vi "CNC.vi"(6 "pause":bool, 7 "start":bool, 8 "products in":u16, 9 "speed in":i32(listbox), 10 "Thermometer in":dbl(slide) scale=0.0..100.0, 11 "speed in":dbl(knob) scale=0.0..10.0) -> (0 "products out":u16, 2 "Thermometer out":dbl(slide) scale=0.0..100.0, 3 "speed out":dbl(knob) scale=0.0..10.0)   [LabVIEW 2026]
uses:
  <vilib>/numeric/Random Number (Range) DBL.vi
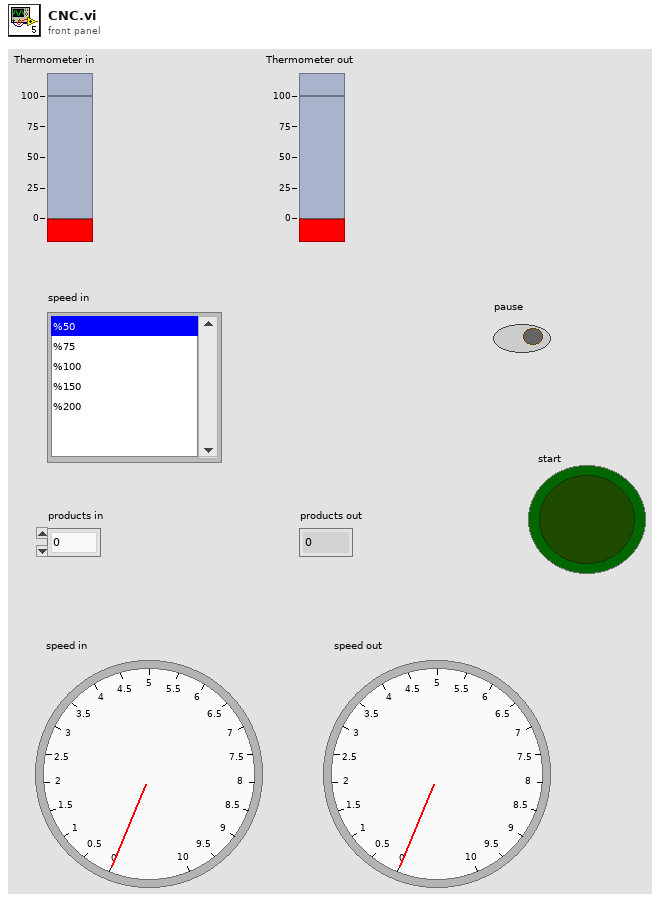
[diagram p1: front panel]
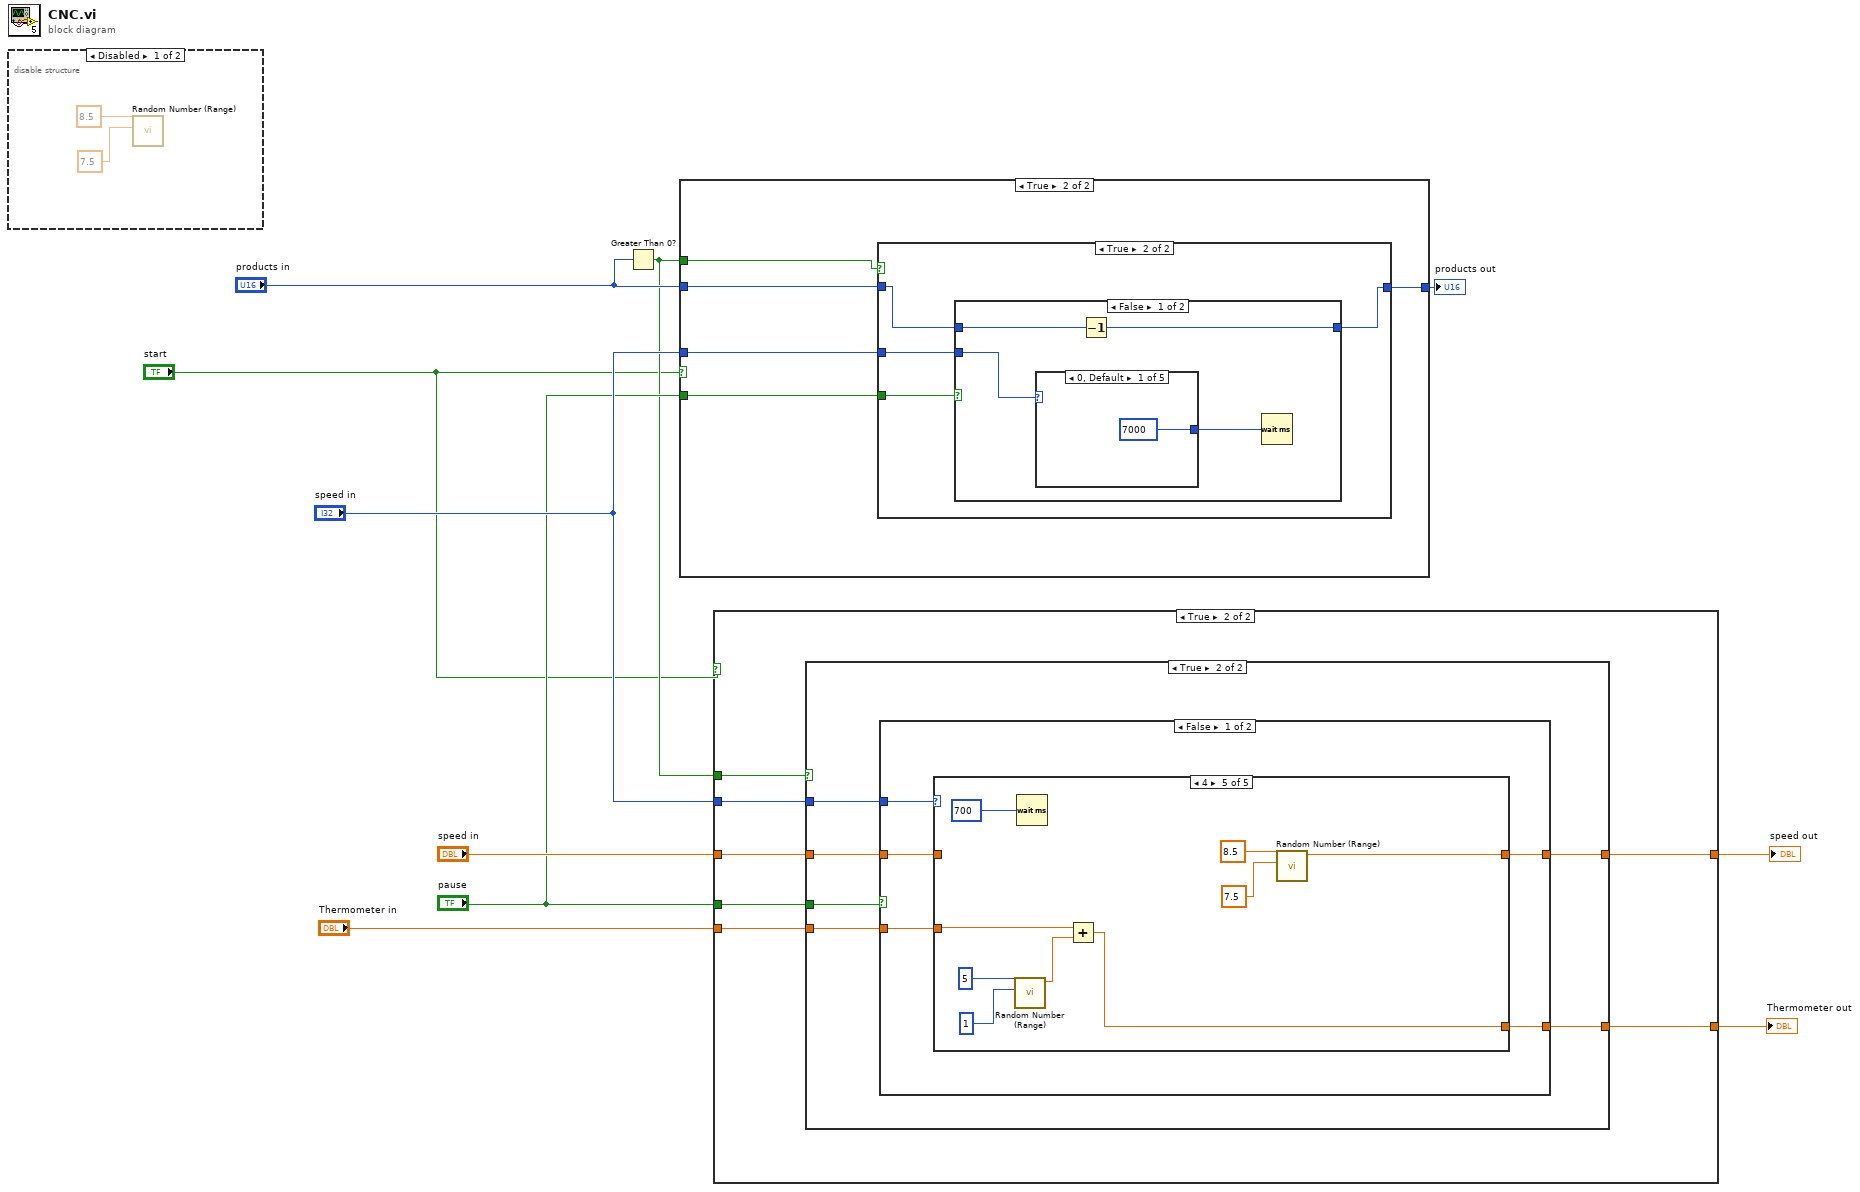
[diagram p0: block diagram]
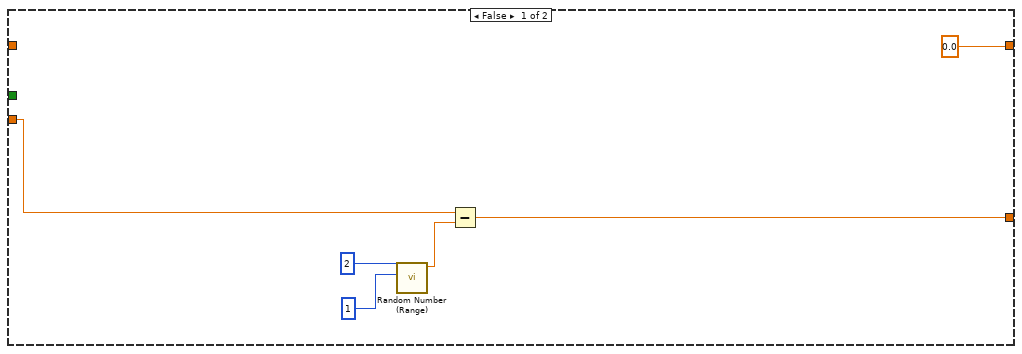
[diagram p2: hidden frame]
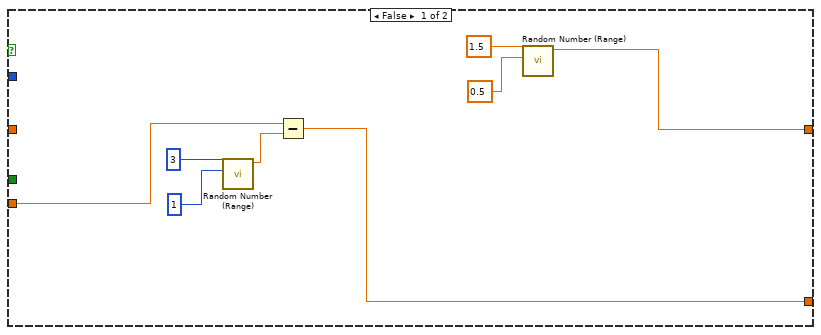
[diagram p3: hidden frame]
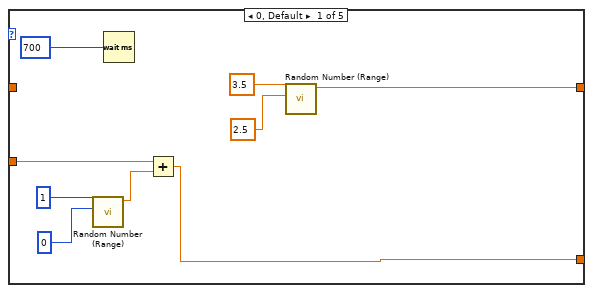
[diagram p4: hidden frame]
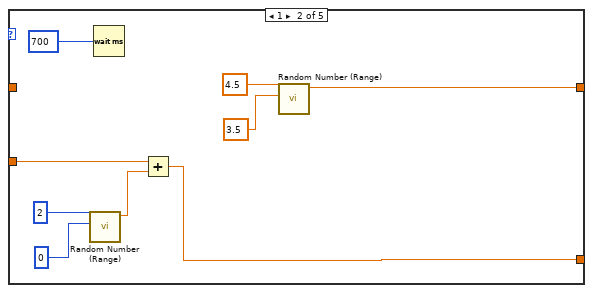
[diagram p5: hidden frame]
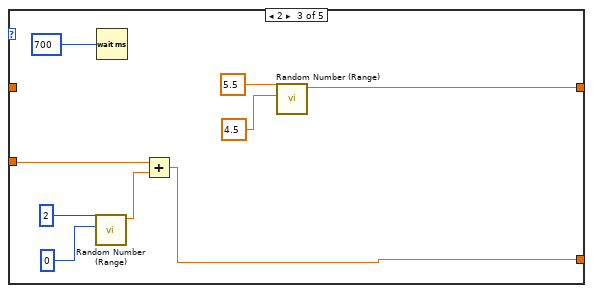
[diagram p6: hidden frame]
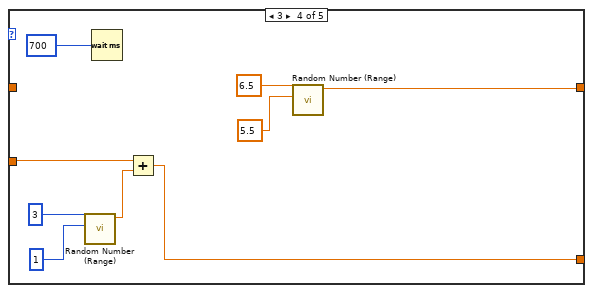
[diagram p7: hidden frame]
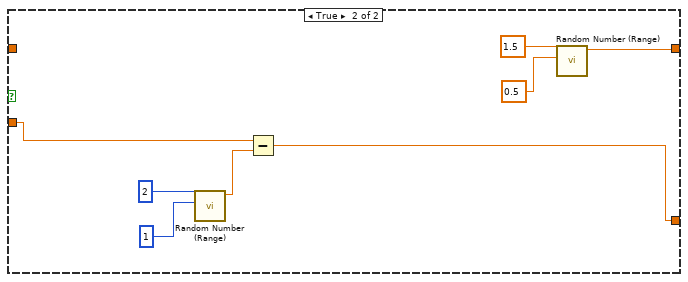
[diagram p8: hidden frame]
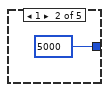
[diagram p11: hidden frame]
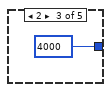
[diagram p12: hidden frame]
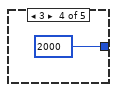
[diagram p13: hidden frame]
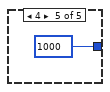
[diagram p14: hidden frame]
diagram:
  n1 = disable-structure shown="Disabled" {
    frame Disabled {
      n2 = call-poly <vilib>:"Random Number (Range).vi"("lower bound (0)"=7.5, "upper bound (100)"=8.5) -> ()  [unwired: 9 in, 1 out]
    }
    frame Enabled {
    }
  }
  n3 = Greater Than 0?(x="products in") -> (x > 0?=w2:bool)
  n4 = case shown="True" "start" {
    tunnel: "products in" -> [w13 w18]
    tunnel: [w13 w17] -> w9
    tunnel: "speed in" -> [_ w16]
    tunnel: "pause" -> [_ w15]
    tunnel: w2 -> [_ w14]
    frame False {
    }
    frame True {
      n5 = case shown="True" w14 {
        tunnel: w18 -> [w19 w22]
        tunnel: [w19 w21] -> w17
        tunnel: w16 -> [_ w23]
        tunnel: w15 -> [_ w20]
        frame False {
        }
        frame True {
          n6 = case shown="False" w20 {
            tunnel: w23 -> [w26 _]
            tunnel: w22 -> [w25 w33]
            tunnel: [w24 w33] -> w21
            frame False {
              n7 = case shown="0, Default" w26 {
                tunnel: [7000 5000 4000 2000 1000] -> w27
                frame 0, Default {
                }
                frame 1 {
                }
                frame 2 {
                }
                frame 3 {
                }
                frame 4 {
                }
              }
              n8 = Decrement(x=w25) -> (x-1=w24:u16)
              n9 = Wait (ms)(milliseconds to wait=w27) -> ()  [unwired: 1 out]
            }
            frame True {
            }
          }
        }
      }
    }
  }
  "products out" <- w9
  n10 = case shown="True" "start" {
    tunnel: "speed in" -> [_ w46]
    tunnel: "Thermometer in" -> [w35 w45]
    tunnel: [w34 w44] -> w6
    tunnel: [0.0 ("speed in") w43] -> w5
    tunnel: "speed in" -> [_ w42]
    tunnel: "pause" -> [_ w41]
    tunnel: w2 -> [_ w40]
    frame False {
      n11 = call-poly <vilib>:"Random Number (Range).vi"("lower bound (0)"=1, "upper bound (100)"=2) -> ("number"=w38:dbl)  [unwired: 9 in]
      n12 = Subtract(x=w35, y=w38) -> (x-y=w34:dbl)
    }
    frame True {
      n13 = case shown="True" w40 {
        tunnel: w46 -> [_ w60]
        tunnel: w45 -> [w51 w59]
        tunnel: [w50 w58] -> w44
        tunnel: [w47 w57] -> w43
        tunnel: w42 -> [_ w56]
        tunnel: w41 -> [_ w55]
        frame False {
          n14 = call-poly <vilib>:"Random Number (Range).vi"("lower bound (0)"=1, "upper bound (100)"=3) -> ("number"=w54:dbl)  [unwired: 9 in]
          n15 = Subtract(x=w51, y=w54) -> (x-y=w50:dbl)
          n16 = call-poly <vilib>:"Random Number (Range).vi"("lower bound (0)"=0.5, "upper bound (100)"=1.5) -> ("number"=w47:dbl)  [unwired: 9 in]
        }
        frame True {
          n17 = case shown="False" w55 {
            tunnel: w60 -> [w65 _]
            tunnel: w59 -> [w64 w112]
            tunnel: [w63 w111] -> w58
            tunnel: [w62 w116] -> w57
            tunnel: w56 -> [w61 _]
            frame False {
              n18 = case shown="4" w65 {
                tunnel: w64 -> [w71 w80 w89 w98 w107]
                tunnel: [w70 w79 w88 w97 w106] -> w63
                tunnel: [w66 w75 w84 w93 w102] -> w62
                tunnel: w61 -> [_ _ _ _ _]
                frame 0, Default {
                  n19 = call-poly <vilib>:"Random Number (Range).vi"("lower bound (0)"=0, "upper bound (100)"=1) -> ("number"=w72:dbl)  [unwired: 9 in]
                  n20 = Wait (ms)(milliseconds to wait=u32 700) -> ()  [unwired: 1 out]
                  n21 = Add(x=w71, y=w72) -> (x+y=w70:dbl)
                  n22 = call-poly <vilib>:"Random Number (Range).vi"("lower bound (0)"=2.5, "upper bound (100)"=3.5) -> ("number"=w66:dbl)  [unwired: 9 in]
                }
                frame 1 {
                  n23 = call-poly <vilib>:"Random Number (Range).vi"("lower bound (0)"=0, "upper bound (100)"=2) -> ("number"=w81:dbl)  [unwired: 9 in]
                  n24 = Wait (ms)(milliseconds to wait=u32 700) -> ()  [unwired: 1 out]
                  n25 = Add(x=w80, y=w81) -> (x+y=w79:dbl)
                  n26 = call-poly <vilib>:"Random Number (Range).vi"("lower bound (0)"=3.5, "upper bound (100)"=4.5) -> ("number"=w75:dbl)  [unwired: 9 in]
                }
                frame 2 {
                  n27 = call-poly <vilib>:"Random Number (Range).vi"("lower bound (0)"=0, "upper bound (100)"=2) -> ("number"=w90:dbl)  [unwired: 9 in]
                  n28 = Wait (ms)(milliseconds to wait=u32 700) -> ()  [unwired: 1 out]
                  n29 = Add(x=w89, y=w90) -> (x+y=w88:dbl)
                  n30 = call-poly <vilib>:"Random Number (Range).vi"("lower bound (0)"=4.5, "upper bound (100)"=5.5) -> ("number"=w84:dbl)  [unwired: 9 in]
                }
                frame 3 {
                  n31 = call-poly <vilib>:"Random Number (Range).vi"("lower bound (0)"=1, "upper bound (100)"=3) -> ("number"=w99:dbl)  [unwired: 9 in]
                  n32 = Wait (ms)(milliseconds to wait=u32 700) -> ()  [unwired: 1 out]
                  n33 = Add(x=w98, y=w99) -> (x+y=w97:dbl)
                  n34 = call-poly <vilib>:"Random Number (Range).vi"("lower bound (0)"=5.5, "upper bound (100)"=6.5) -> ("number"=w93:dbl)  [unwired: 9 in]
                }
                frame 4 {
                  n35 = call-poly <vilib>:"Random Number (Range).vi"("lower bound (0)"=1, "upper bound (100)"=5) -> ("number"=w110:dbl)  [unwired: 9 in]
                  n36 = Wait (ms)(milliseconds to wait=u32 700) -> ()  [unwired: 1 out]
                  n37 = Add(x=w107, y=w110) -> (x+y=w106:dbl)
                  n38 = call-poly <vilib>:"Random Number (Range).vi"("lower bound (0)"=7.5, "upper bound (100)"=8.5) -> ("number"=w102:dbl)  [unwired: 9 in]
                }
              }
            }
            frame True {
              n39 = call-poly <vilib>:"Random Number (Range).vi"("lower bound (0)"=1, "upper bound (100)"=2) -> ("number"=w115:dbl)  [unwired: 9 in]
              n40 = Subtract(x=w112, y=w115) -> (x-y=w111:dbl)
              n41 = call-poly <vilib>:"Random Number (Range).vi"("lower bound (0)"=0.5, "upper bound (100)"=1.5) -> ("number"=w116:dbl)  [unwired: 9 in]
            }
          }
        }
      }
    }
  }
  "Thermometer out" <- w6
  "speed out" <- w5
